vi "Get Tolerance Val (SubVI).vi"(10 "Tolerance":u16) -> (2 "Tolerance Value":dbl)   [LabVIEW 2011]
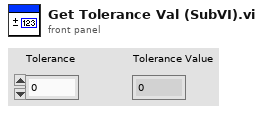
[diagram p1: front panel]
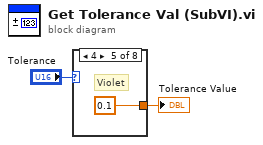
[diagram p0: block diagram]
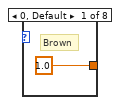
[diagram p2: hidden frame]
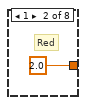
[diagram p3: hidden frame]
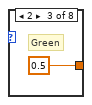
[diagram p4: hidden frame]
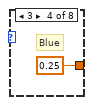
[diagram p5: hidden frame]
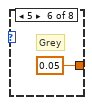
[diagram p6: hidden frame]
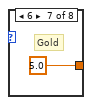
[diagram p7: hidden frame]
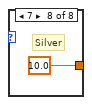
[diagram p8: hidden frame]
diagram:
  n1 = case shown="4" "Tolerance" {
    tunnel: [1.0 2.0 0.5 0.25 0.1 0.05 5.0 10.0] -> w2
    frame 0, Default {
      # "Brown"
    }
    frame 1 {
      # "Red"
    }
    frame 2 {
      # "Green"
    }
    frame 3 {
      # "Blue"
    }
    frame 4 {
      # "Violet"
    }
    frame 5 {
      # "Grey"
    }
    frame 6 {
      # "Gold"
    }
    frame 7 {
      # "Silver"
    }
  }
  "Tolerance Value" <- w2
